vi "Run.vi"   [LabVIEW 2016, in "TriggerAction Q.lvclass"]
uses:
  <userlib>/Common Components/TriggerAction Q/TriggerAction Q/TriggerAction Q.lvclass
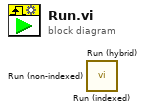
[diagram p0: block diagram]
diagram:
  n1 = call <userlib>:"Run (hybrid).vi"() -> ()  [unwired: 10 in, 2 out]
  n2 = call <userlib>:"Run (indexed).vi"() -> ()  [unwired: 10 in, 2 out]
  n3 = call <userlib>:"Run (non-indexed).vi"() -> ()  [unwired: 10 in, 2 out]
